vi "Get Strings from Enum__ogtk.vi"(8 "error in (no error)":errorcluster, 10 "Enum":variant) -> (0 "error out":errorcluster, 1 "String Value":string, 2 "Enum Strings":string[](array[string]), 3 "Enum Name":string)   [LabVIEW 2023, in "openg_variant.lvlib"]
doc: "Returns Enum Strings array, String Value and Enum Name from an Enum."
uses:
  openg_variant.lvlib
  error/error.llb/openg_error.lvlib
panel:
  # "[OpenG VI Tags] ***Do Not Remove***"
  # "Get Strings from Enum.vi\n\nReturns Enum Strings array, String Value and Enum Name from an Enum.\n\nPlease visit http://www.OpenG.org to learn about the\nOpen Source LabVIEW software movement.\n\nNOTICE -- YOU MUST LEAVE THIS NOTICE IN PLACE.  PER THE TERMS OF THE LICENSE BELOW, YOU MAY SUBLICENSE THIS SOFTWARE \nIN ANY WAY THAT DOES NOT CONFLICT WITH THIS LICENSE.\n\n### BSD License (http://www.opensource.org/licenses/bsd-license.php) Begin ###\n \nCopyright (c) 2002, Jean-Pierre Drolet <drolet_jp@hotmail.com>\nCopyright (c) 2002-2006, Jim Kring <jim@jimkring.com>\n\nAll rights reserved.\n\nRedistribution and use in source and binary forms, with or without modification, are permitted provided that the following conditions are met:\n\n    * Redistributions of source code must retain the above copyright notice, this list of conditions and the following disclaimer.\n    * Redistributions in binary form must reproduce the above copyright notice, this list of conditions and the following disclaimer in the \n       documentation and/or other materials provided with the distribution.\n    * Neither the name of SciWare, James Kring, Inc., nor the names of its contributors may be used to endorse or promote products derived \n       from this software without specific prior written permission.\n\nTHIS SOFTWARE IS PROVIDED BY THE COPYRIGHT HOLDERS AND CONTRIBUTORS \"AS IS\" AND ANY EXPRESS OR IMPLIED WARRANTIES, \nINCLUDING, BUT NOT LIMITED TO, THE IMPLIED WARRANTIES OF MERCHANTABILITY AND FITNESS FOR A PARTICULAR PURPOSE ARE \nDISCLAIMED. IN NO EVENT SHALL THE COPYRIGHT OWNER OR CONTRIBUTORS BE LIABLE FOR ANY DIRECT, INDIRECT, INCIDENTAL,\n SPECIAL, EXEMPLARY, OR CONSEQUENTIAL DAMAGES (INCLUDING, BUT NOT LIMITED TO, PROCUREMENT OF SUBSTITUTE GOODS OR \nSERVICES; LOSS OF USE, DATA, OR PROFITS; OR BUSINESS INTERRUPTION) HOWEVER CAUSED AND ON ANY THEORY OF LIABILITY, \nWHETHER IN CONTRACT, STRICT LIABILITY, OR TORT (INCLUDING NEGLIGENCE OR OTHERWISE) ARISING IN ANY WAY OUT OF THE USE \nOF THIS SOFTWARE, EVEN IF ADVISED OF THE POSSIBILITY OF SUCH DAMAGE.\n\n### BSD License End ###"
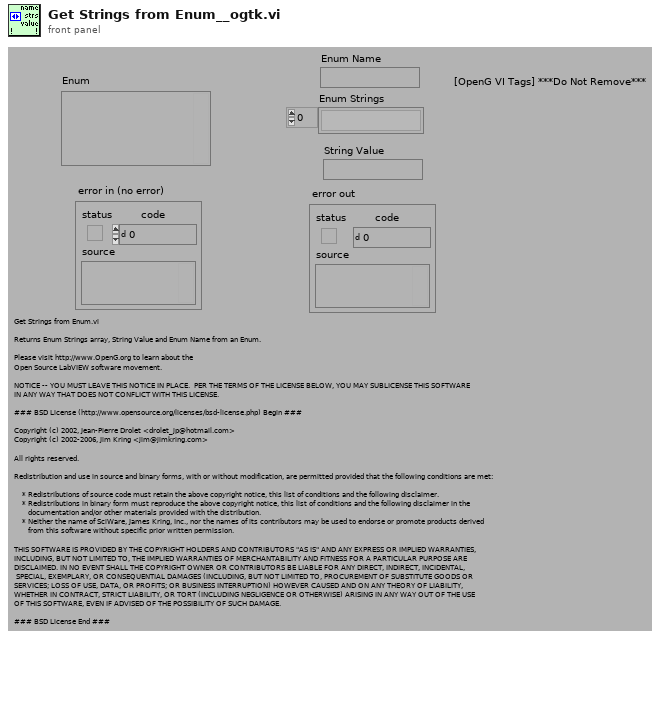
[diagram p1: front panel]
types:
  T1 = typedef "openg_variant.lvlib/Type Descriptor Header__ogtk.ctl" = cluster{"length":u16, "private":u8, "type":T2, "# elements":u16}
  T2 = typedef "openg_variant.lvlib/Type Descriptor Enumeration__ogtk.ctl" = enum8{"<Null>", "I8", "I16", "I32", "I64", "U8", "U16", "U32", "U64", "SGL", "DBL", "EXT", "CSG", "CDB", "CXT", "0x0F", "0x10", "0x11", "0x12", "0x13", "0x14", "Enum U8", "Enum U16", "Enum U32", "Enum U64", "SGL PQ", "DBL PQ", "EXT PQ", "CSG PQ", "CDB PQ", "CXT PQ", "0x1F", "0x20", "Boolean", "0x22", "0x23", "0x24", "0x25", "0x26", "0x27", "0x28", "0x29", "0x2A", "0x2B", "0x2C", "0x2D", "0x2E", "0x2F", "String", "0x31", "Path", "Pict", "0x34", "0x35", "0x36", "DAQ", "0x38", "0x39", "0x3A", "0x3B", "0x3C", "0x3D", "0x3E", "0x3F", "Array", "0x41", "0x42", "0x43", "0x44", "0x45", "0x46", "0x47", "0x48", "0x49", "0x4A", "0x4B", "0x4C", "0x4D", "0x4E", "0x4F", "Cluster", "0x51", "0x52", "Variant", "Waveform", "0x55", "0x56", "0x57", "0x58", "0x59", "0x5A", "0x5B", "0x5C", "0x5D", "0x5E", "Fixed Point", "0x60", "0x61", "0x62", "0x63", "0x64", "0x65", "0x66", "0x67", "0x68", "0x69", "0x6A", "0x6B", "0x6C", "0x6D", "0x6E", "0x6F", "Refnum", "0x71", "0x72", "Set Collection", "Map Collection"}
  T3 = typedef "openg_variant.lvlib/Type Descriptor__ogtk.ctl" = i16[]
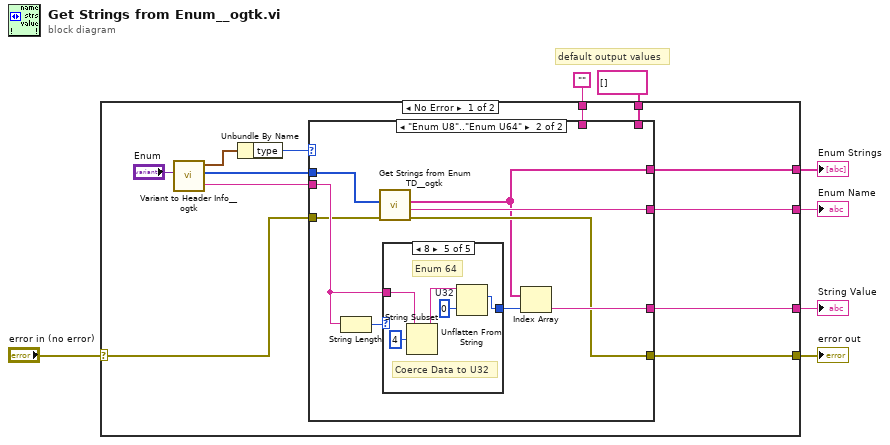
[diagram p0: block diagram]
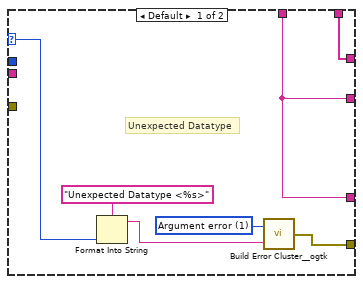
[diagram p2: hidden frame]
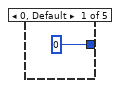
[diagram p3: hidden frame]
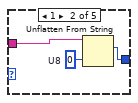
[diagram p4: hidden frame]
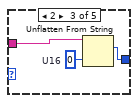
[diagram p5: hidden frame]
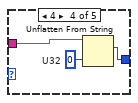
[diagram p6: hidden frame]
diagram:
  # "default output values"
  n1 = case shown="No Error" "error in (no error)" {
    selector: "error in (no error)" -> [w10 w53]
    tunnel: [w19 w53] -> w7
    tunnel: [w13 w52] -> w5
    tunnel: [w12 w51] -> w4
    tunnel: [w11 w51] -> w3
    tunnel: string[] [] -> [w9 w52]
    tunnel: "" -> [w8 w51]
    frame No Error {
      n2 = call "Variant to Header Info__ogtk.vi"("Variant"="Enum") -> ("Type Descriptor Header"=w18:T1, "Type Descriptor"=w15:T3, "data string"=w14:string)  [unwired: 3 in]
      n3 = Unbundle By Name(w18) -> ("type"=w17:T2)
      n4 = case shown="\"Enum U8\"..\"Enum U64\"" w17 {
        selector: w17 -> [w25 _]
        tunnel: [w22 w28] -> w19
        tunnel: w15 -> [_ w30]
        tunnel: w14 -> [_ w34]
        tunnel: [w21 w27] -> w13
        tunnel: [w20 w31] -> w12
        tunnel: [w20 w32] -> w11
        tunnel: w10 -> [_ w29]
        tunnel: w9 -> [w21 _]
        tunnel: w8 -> [w20 _]
        frame Default {
          w26 = 1 items=["No error", "Argument error", "Memory is full", "Out of zone", "End of file", "File already open", "Generic file I/O error", "File not found", "File permission error", "Disk is full", "Duplicate path", "Too many files open", "System feature not enabled", "Resource file not found", "Cannot add resource", "Resource not found", "Image not found", "Image memory error", "Pen does not exist", "Config type invalid", "Config token not found", "Config parse error", "Config memory error", "Bad external code format", "Bad external code offset", "External code not present", "Null window", "Destroy window error", "Null menu", "Print aborted", "Bad print record", "Print driver error", "Windows error during printing", "Memory error during printing", "Print dialog error", "Generic print error", "Invalid device refnum", "Device not found", "Device parameter error", "Device unit error", "Cannot open device", "Device call aborted", "Generic error", "Cancelled by user", "Object ID too low", "Object ID too high", "Object not in heap", "Unknown heap", "Unknown object (invalid DefProc)", "Unknown object (DefProc not in table)", "Message out of range", "Invalid (null) method", "Unknown message", "Manager call not supported", "Bad address", "Network operation in progress", "Network operation timed out", "Connection is busy", "Network attribute not supported", "Network error", "Address in use", "System out of memory", "Connection aborted", "Connection refused", "Not connected", "Already connected", "Connection closed", "Initialization error (interapplication manager)", "Bad occurrence", "Wait on unbound occurrence handler", "Occurrence queue overflow", "Datalog type conflict", "Unused", "Unrecognized type (interapplication manager)", "Memory corrupt", "Failed to make temporary DLL", "Old CIN version", "Drag socket not found", "Failed to load drop-object", "Failed to register OLE object", "Failed to release OLE object", "Format specifier type mismatch", "Unknown format specifier", "Too few format specifiers", "Too many format specifiers", "Scan failed", "Newer CIN version", "Error converting to variant", "Runtime menu error", "Password tampered", "Variant attribute not found", "Incompatible variant data type", "Event data is not available", "Event Store is not present", "Occurrence is not found", "Event Queue is not created", "Event info is not available", "Refnum passed is NULL", "Error retrieving Class GUID", "Error retrieving CoClass GUID", "Error retrieving TypeLib GUID.", "Bad built application magic bytes.", "Specific driver is different from the specific driver associated with the Logical Name.", "There is no session opened to the class driver.", "Max Error", "MAX - Error with config objects", "MAX - Error loading configuration", "MAX - Group not supported"]
          # "Unexpected Datatype"
          n5 = Format Into String(format string="Unexpected Datatype <%s>" ("Format String"), w25) -> (resulting string=w23:string)  [unwired: 2 in, 1 out]
          n6 = call "Build Error Cluster__ogtk.vi"("String to Prepend to source (\"\")"=w23, "code"=w26) -> ("error out"=w22:errorcluster)
        }
        frame "Enum U8".."Enum U64" {
          n7 = String Length(string=w34) -> (length=w35:i32)
          n8 = call "Get Strings from Enum TD__ogtk.vi"("error in (no error)"=w29, "Type Descriptor"=w30) -> ("error out"=w28:errorcluster, "enum name"=w31:string, "enum strings"=w27:string[])  [unwired: 7 in]
          n9 = case shown="8" w35 {
            tunnel: w34 -> [_ w39 w42 w45 w46]
            tunnel: [u32 0 ("U32") w37 w40 w43 w49] -> w33
            frame 0, Default {
            }
            frame 1 {
              w38 = u8 0  # U8
              n10 = Unflatten From String(type=w38, binary string=w39) -> (value=w37:u8)  [unwired: 3 in, 2 out]
            }
            frame 2 {
              w41 = u16 0  # U16
              n11 = Unflatten From String(type=w41, binary string=w42) -> (value=w40:u16)  [unwired: 3 in, 2 out]
            }
            frame 4 {
              w44 = u32 0  # U32
              n12 = Unflatten From String(type=w44, binary string=w45) -> (value=w43:u32)  [unwired: 3 in, 2 out]
            }
            frame 8 {
              w50 = u32 0  # U32
              # "Coerce Data to U32"
              # "Enum 64"
              n13 = String Subset(string=w46, offset (0)=4) -> (substring=w47:string)  [unwired: 1 in]
              n14 = Unflatten From String(type=w50, binary string=w47) -> (value=w49:u32)  [unwired: 3 in, 2 out]
            }
          }
          n15 = Index Array(array=w27, index=w33) -> (element=w32:string)
        }
      }
    }
    frame Error {
    }
  }
  "error out" <- w7
  "Enum Strings" <- w5
  "Enum Name" <- w4
  "String Value" <- w3
